vi "GMLAN RequestDownload.vi"(7 "unCompressedMemorySize Length":enum8{"Two", "Three", "Four"}(ring), 8 "error in (no error)":errorcluster, 9 "dataFormatIdentifier":u8 format="%.0b", 10 "unCompressedMemorySize":u32, 11 "diag ref in":T1) -> (0 "error out":errorcluster, 1 "success?":bool, 3 "diag ref out":T1)   [LabVIEW 2015, in "GMLAN.lvlib"]
uses:
  GMLAN.lvlib
  <vilib>/Automotive Diagnostic Command Set/Diagnostic Transport.llb/Diag Reference.ctl
  <vilib>/Automotive Diagnostic Command Set/Diagnostic Transport.llb/Transport Protocol Selector.ctl
  <vilib>/Automotive Diagnostic Command Set/Diagnostic Transport.llb/Diag CAN Frame Log.ctl
  <vilib>/addons/Automotive Diagnostic Command Set/NI_Automotive Diagnostic Command Set.lvlib
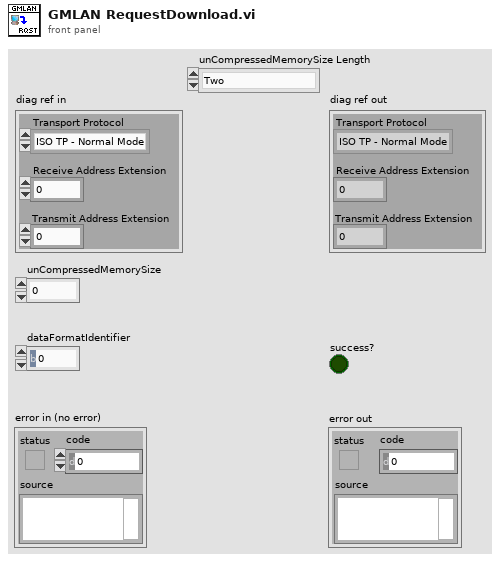
[diagram p1: front panel]
types:
  T1 = typedef "NI_Automotive Diagnostic Command Set.lvlib/Diag Reference.ctl" = cluster{"Diag CAN Handle":u32, "Transport Protocol":T2, "Receive Address Extension":u8, "Transmit Address Extension":u8, "Receive CAN Id":u32, "Transmit CAN Id":u32, "Diag CAN Queue":refnum<queue>, "Log Frames ?":bool, "My TP Address":u8, "Other TP Address":u8, "T1":u16, "T2":u16, "T3":u16, "T4":u16, "Tx SN":u8, "Block Size":u8, "Rx SN":u8, "VW TP Initialized?":bool, "Tx block no":u8, "baud rate":u32, "Interface":string, "Channel Diag CAN Handle":u32, "UDP Connection ID":refnum<k16>, "TCP Connection ID":refnum<k5>, "Target IP Addr":u32, "Source Address":u16, "Target Address":u16, "Send Header NACK?":bool, "DLL Handle":u32, "NAD":u8, "Time Stamp read first":dbl, "Time Stamp read last":dbl, "Time Stamp write first":dbl, "Time Stamp write last":dbl, "Time Stamp write":dbl, "Time Stamp read":dbl}
  T2 = typedef "NI_Automotive Diagnostic Command Set.lvlib/Transport Protocol Selector.ctl" = enum16{"ISO TP - Normal Mode", "ISO TP - Mixed Mode", "VW TP 2.0", "Diagnostics on IP", "ISO TP LIN"}
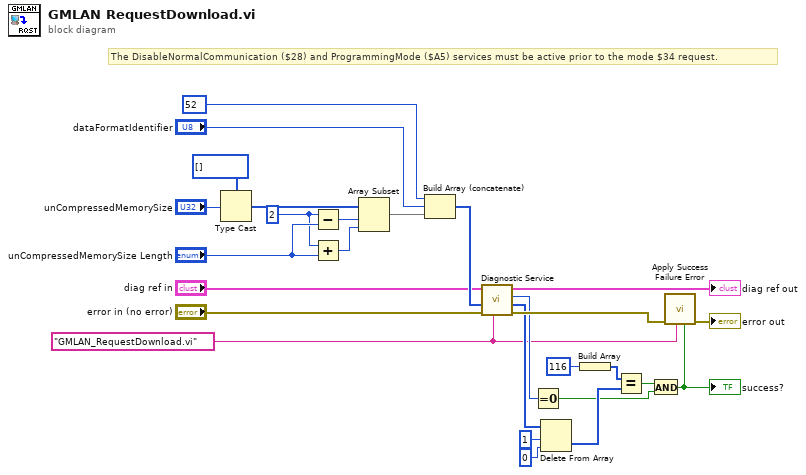
[diagram p0: block diagram]
diagram:
  w5 = 2 ("index")
  w11 = "GMLAN_RequestDownload.vi" ("error source")
  # "The DisableNormalCommunication ($28) and ProgrammingMode ($A5) services must be active prior to the mode $34 request."
  n1 = Type Cast(type=u8[] [], x="unCompressedMemorySize") -> (*(type *) &x=w8:u8[])
  n2 = Subtract(x=w5, y="unCompressedMemorySize Length") -> (x-y=w6:i32)
  n3 = Add(x=w5, y="unCompressedMemorySize Length") -> (x+y=w4:i32)
  n4 = Array Subset(array=w8, index=w6, length=w4) -> (w3:u8[])
  n5 = Build Array (concatenate)(u8 52 ("element"), "dataFormatIdentifier", w3) -> (w23:u8[])
  n6 = call <vilib>:"Diagnostic Service.vi"("error source"=w11, "error in (no error)"="error in (no error)", "data in"=w23, "diag ref in"="diag ref in") -> ("error out"=w25:errorcluster, "data out"=w18:u8[], "error code"=w22:u8, "diag ref out"=→"diag ref out":T1)  [unwired: 2 in, 2 out]
  n7 = Equal To 0?(x=w22) -> (x = 0?=w16:bool)
  n8 = Delete From Array(array=w18, length=1, index=0) -> (deleted portion=w17:u8[])  [unwired: 1 out]
  n9 = Build Array(u8 116 ("element")) -> (w19:u8[])
  n10 = Equal?(x=w19, y=w17) -> (x = y?=w15:bool)
  n11 = And(x=w15, y=w16) -> (x .and. y?=w12:bool)
  "success?" <- w12
  n12 = call <vilib>:"Apply Success Failure Error.vi"("success code"=w12, "error source"=w11, "error in (no error)"=w25) -> ("error out"=→"error out":errorcluster)  [unwired: 8 out]
